vi "Read Categories.vi"(8 "error in (no error)":errorcluster, 11 "StoreUI in":refnum<class "StoreUI.lvclass">) -> (0 "error out":errorcluster, 2 "Categories":refnum<data-value>, 3 "StoreUI out":refnum<class "StoreUI.lvclass">)   [LabVIEW 2015]
uses:
  StoreUI.lvclass
  Classes/Category/Category.lvclass
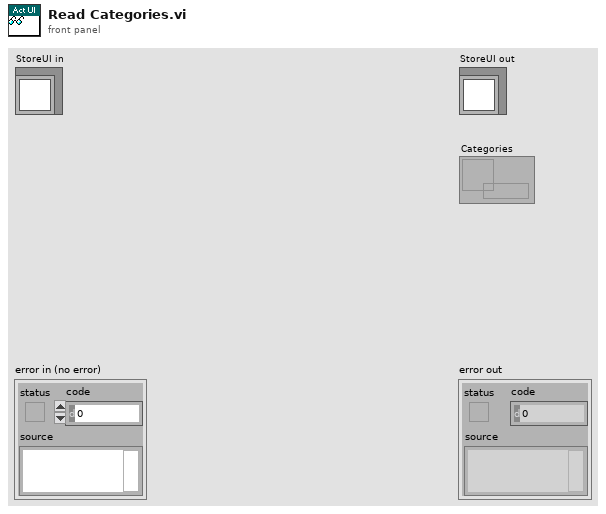
[diagram p1: front panel]
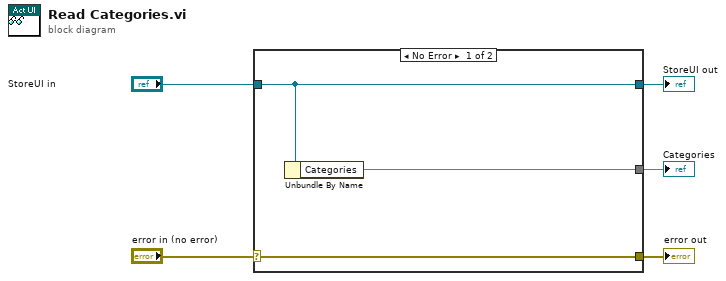
[diagram p0: block diagram]
diagram:
  n1 = case shown="No Error" "error in (no error)" {
    selector: "error in (no error)" -> [w8 w9]
    tunnel: [w8 w9] -> w4
    tunnel: [w7 w10] -> w2
    tunnel: "StoreUI in" -> [w7 w10]
    tunnel: [w6 _] -> w1
    frame No Error {
      n2 = Unbundle By Name(w7) -> ("Categories"=w6)
    }
    frame Error {
    }
  }
  "error out" <- w4
  "StoreUI out" <- w2
  "Categories" <- w1
